vi "Disc_Teleop.vi"(1 "Joystick_Out":T1) -> ()   [LabVIEW 2018]
uses:
  Utility_VIs/Joystick_Controls.ctl
  Subsytems/Intake_Disc/Intake_Disc_Notifier.ctl
  Subsytems/Intake_Disc/Intake_Disc_Control_Type.ctl
  <vilib>/Rock Robotics/WPI/Solenoid/WPI_SolenoidValue.ctl
  Global_Variables/Intake_Disc_Globals.vi
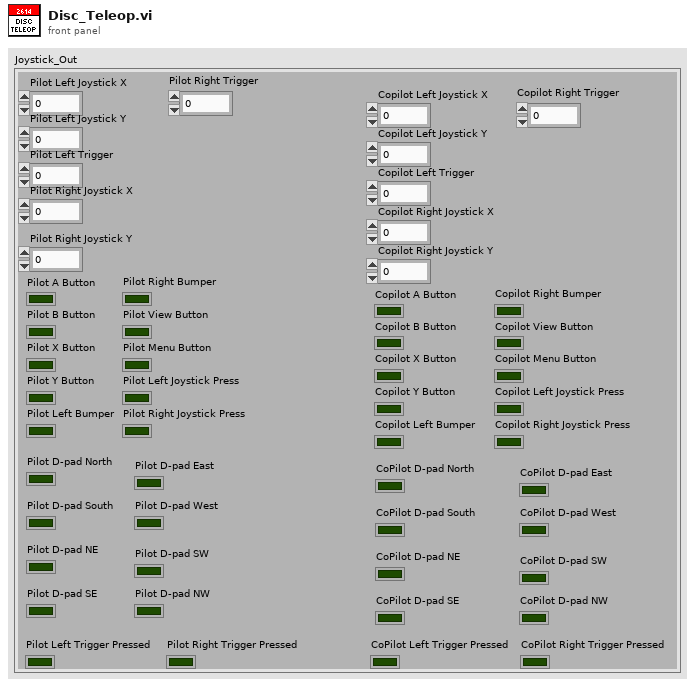
[diagram p1: front panel]
types:
  T1 = typedef "Joystick_Controls.ctl" = cluster{"Pilot Left Joystick X":dbl, "Pilot Left Joystick Y":dbl, "Pilot A Button":bool, "Pilot B Button":bool, "Pilot X Button":bool, "Pilot Y Button":bool, "Pilot Left Bumper":bool, "Pilot Right Bumper":bool, "Pilot View Button":bool, "Pilot Menu Button":bool, "Pilot Left Joystick Press":bool, "Pilot Right Joystick Press":bool, "Pilot Left Trigger":dbl, "Pilot Right Joystick X":dbl, "Pilot Right Joystick Y":dbl, "Pilot Right Trigger":dbl, "Copilot Left Joystick X":dbl, "Copilot Left Joystick Y":dbl, "Copilot A Button":bool, "Copilot B Button":bool, "Copilot X Button":bool, "Copilot Y Button":bool, "Copilot Left Bumper":bool, "Copilot Right Bumper":bool, "Copilot View Button":bool, "Copilot Menu Button":bool, "Copilot Left Joystick Press":bool, "Copilot Right Joystick Press":bool, "Copilot Left Trigger":dbl, "Copilot Right Joystick X":dbl, "Copilot Right Joystick Y":dbl, "Copilot Right Trigger":dbl, "Pilot D-pad North":bool, "Pilot D-pad South":bool, "Pilot D-pad East":bool, "Pilot D-pad West":bool, "Pilot D-pad NE ":bool, "Pilot D-pad SE":bool, "Pilot D-pad SW":bool, "Pilot D-pad NW":bool, "CoPilot D-pad North":bool, "CoPilot D-pad South":bool, "CoPilot D-pad East":bool, "CoPilot D-pad West":bool, "CoPilot D-pad NE":bool, "CoPilot D-pad SE":bool, "CoPilot D-pad SW":bool, "CoPilot D-pad NW":bool, "Pilot Left Trigger Pressed":bool, "Pilot Right Trigger Pressed":bool, "CoPilot Left Trigger Pressed":bool, "CoPilot Right Trigger Pressed":bool}
  T2 = typedef "Intake_Disc_Notifier.ctl" = cluster{"Intake_Disc_Control_Type":T3, "Manual_Disc_Toggle":bool, "Disc_Toggle":bool, "Disc_Toggle_State":bool, "Manual_Press_Toggle":bool, "Disc_Press_State":bool, "Press_Toggle":bool, "Press_Pnuematic":T4, "Disc_Pnuematic":T4, "Disc_Notifier":refnum<notifier>, "Step":i32}
  T3 = typedef "Intake_Disc_Control_Type.ctl" = enum16{"No_Op", "Manual_Disc_Toggle", "Disc_Toggle", "Manual_Press_Toggle", "Press_Toggle", "Acquire_Hatch", "Retract"}
  T4 = typedef "WPI_SolenoidValue.ctl" = enum16{"Off", "On", "Forward", "Reverse"}
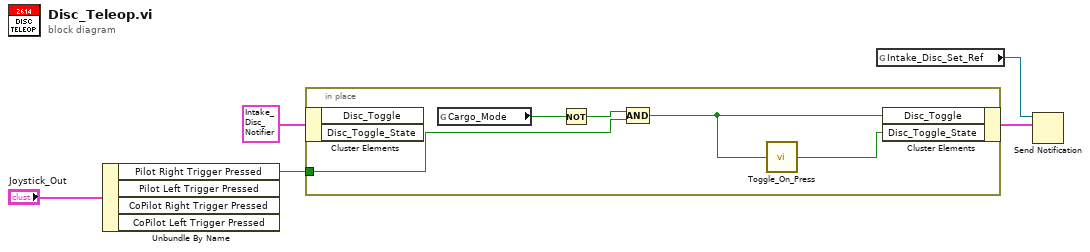
[diagram p0: block diagram]
diagram:
  n1 = Unbundle By Name("Joystick_Out") -> ("Pilot Right Trigger Pressed"=w3:bool)  [unwired: 3 out]
  n2 = in-place {
    in-place-border: w3 -> [w8]
    n3 = in-place-cluster #1(T2 {"Intake_Disc_Control_Type"=enum."No_Op", "Manual_Disc_Toggle"=FALSE, "Disc_Toggle"=FALSE, "Disc_Toggle_State"=FALSE, "Manual_Press_Toggle"=FALSE, "Disc_Press_State"=FALSE, "Press_Toggle"=FALSE, "Press_Pnuematic"=enum."Forward", "Disc_Pnuematic"=enum."Forward", "Disc_Notifier"=refnum, "Step"=0} ("Intake_Disc_Notifier")) -> ()  [unwired: 2 out]
    n4 = global read "Intake_Disc_Globals.vi" "Cargo_Mode"() -> (w10:bool)
    n5 = Not(x=w10) -> (.not. x?=w9:bool)
    n6 = Compound Arithmetic op=AND(w9, w8) -> (w7:bool)
    n7 = call "Toggle_On_Press.vi"("Boolean"=w7) -> ("Boolean Out"=w6:bool)
    n8 = in-place-cluster #1("Disc_Toggle"=w7, "Disc_Toggle_State"=w6) -> (w2:T2)
  }
  n9 = global read "Intake_Disc_Globals.vi" "Intake_Disc_Set_Ref"() -> (w1:refnum<notifier>)
  n10 = Send Notification(notification=w2, notifier=w1) -> ()  [unwired: 1 in, 2 out]
